vi "Cast.vi"(4 "Number of Shifts":i32, 6 "Lookup Table":sgl[](array[numeric]), 7 "Method":T1 items=["Use Bit Depth", "Shift", "Use Lookup Table"], 8 "error in":errorcluster, 9 "Image Type":T2, 10 "Image Dst Reference In":T3, 11 "Image Src Reference In":T3) -> (0 "error out":errorcluster, 3 "Image Dst Reference Out":T3)   [LabVIEW 2024, in "OpenLvVision_Image.lvlib" / "Management.lvlib"]
doc: "Converts the image's pixel data type. \nFor 8-bit and 16-bit images, the scaling method for this conversion is set by the specified \"Method\"."
uses:
  Management.lvlib
  TypeDef/Image.ctl
  TypeDef/ImageType.ctl
  <vilib>/vision/Management.llb/Cast Image 2 Method.ctl
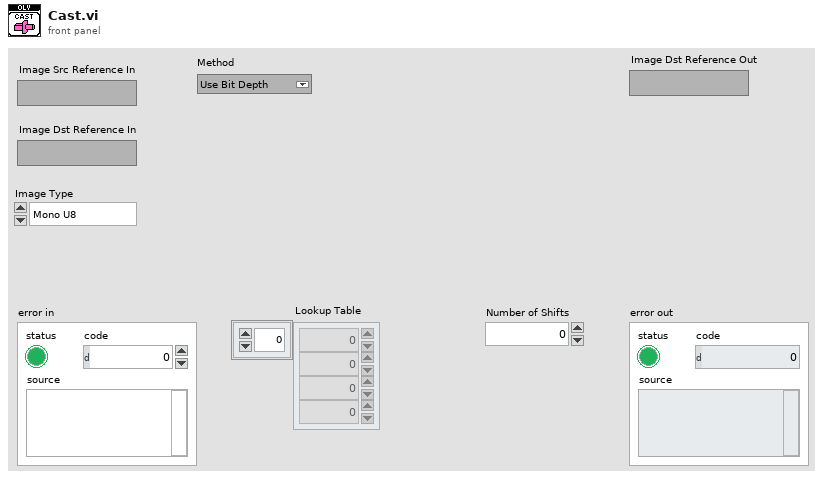
[diagram p1: front panel]
types:
  T1 = typedef "Cast Image 2 Method.ctl" = u32
  T2 = typedef "OpenLvVision_Image.lvlib/Management.lvlib/ImageType.ctl" = enum16{"Mono U8", "Mono U16", "Mono I16", "Mono SGL", "Color U32", "Color U64"}
  T3 = typedef "OpenLvVision_Image.lvlib/Management.lvlib/Image.ctl" = refnum<image>
  T4 = typedef "Image Type" = u32
  T5 = typedef "IMAQ Image.ctl" = refnum<image>
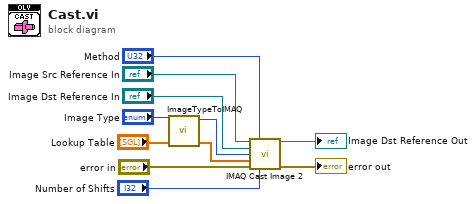
[diagram p0: block diagram]
diagram:
  n1 = call "ImageTypeToIMAQ.vi"("OLV Image Type"="Image Type") -> ("IMAQ Image Type"=w4:T4)  [unwired: 10 in]
  n2 = call "IMAQ Cast Image 2"("Image Src"="Image Src Reference In", "Method"="Method", "Image Dst"="Image Dst Reference In", "Image Type"=w4, "Lookup Table"="Lookup Table", "error in (no error)"="error in", "Number of Shifts"="Number of Shifts") -> ("Image Dst Out"=→"Image Dst Reference Out":T5, "error out"=→"error out":errorcluster)  [unwired: 7 in]
